vi "ethernet bc init.vi"(8 "error in":errorcluster, 10 "remote port or service name":u16, 11 "address":string) -> (0 "error out":errorcluster, 3 "TCP Network Connection out":refnum<k5>)   [LabVIEW 2018]
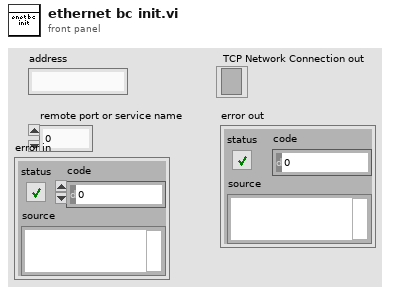
[diagram p1: front panel]
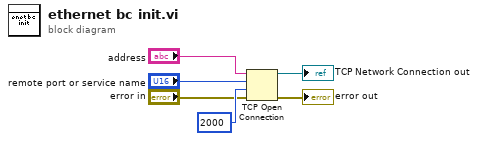
[diagram p0: block diagram]
diagram:
  n1 = TCP Open Connection(address="address", remote port or service name="remote port or service name", timeout ms (60000)=2000, error in (no error)="error in") -> (connection ID=→"TCP Network Connection out":refnum<k5>, error out=→"error out":errorcluster)  [unwired: 1 in]
